vi "Configure Motor Controllers.vi"(8 "error in (no error)":errorcluster, 11 "Motion Magic Parameters":T1) -> (0 "error out":errorcluster)   [LabVIEW 2017, in "Drive Train.lvlib"]
uses:
  Drive Train.lvlib
  Controls/FGV Actions.ctl
  Controls/Motor Controllers Parameters.ctl
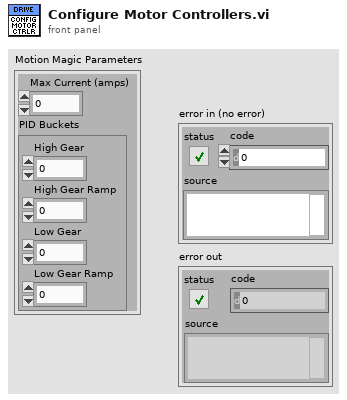
[diagram p1: front panel]
types:
  T1 = typedef "Drive Train.lvlib/Motor Controllers Parameters.ctl" = cluster{"Max Current (amps)":i32, "PID Buckets":cluster{"High Gear":i32, "High Gear Ramp":i32, "Low Gear":i32, "Low Gear Ramp":i32}}
  T2 = typedef "Drive Train.lvlib/FGV Actions.ctl" = enum16{"Get", "Set"}
  T3 = typedef "Drive Train.lvlib/Library Information.ctl" = cluster{"Right Motor Name":string, "Left Motor Name":string, "Current Control Mode":T4, "Motion Magic Parameters":T5, "Motor Controllers Parameters":T1}
  T4 = typedef "CTRE_Phoenix_MotorControl_ControlMode.ctl" = u16
  T5 = typedef "Drive Train.lvlib/Motion Magic Parameters.ctl" = cluster{"Native Units":dbl}
  T6 = typedef "WPI_MotorControlDeviceRef.ctl" = cluster{"DeviceStatus":errorcluster, "Type":T7, "PWM":cluster{"PWM Channel":T8, "DeadBand":T9}, "CAN":cluster{"Device Number":u8, "SetOutput VI Ref":variant, "GetOutput VI Ref":variant, "Enable VI Ref":variant, "Disable VI Ref":variant, "Data":variant}, "Invert":bool, "DIO PWM":cluster{"PWM \"Enable\" Channel":T8, "DIOChannel":T10, "PWM Rate":dbl}}
  T7 = typedef "WPI_MotorControlType.ctl" = enum16{"PWM", "CAN", "DIO PWM"}
  T8 = typedef "FPGA_DIOPWMChannel.ctl" = enum8{"PWM 0", "PWM 1", "PWM 2", "PWM 3", "PWM 4", "PWM 5", "PWM 6", "PWM 7", "PWM 8", "PWM 9", "PWM MXP 0", "PWM MXP 1", "PWM MXP 2", "PWM MXP 3", "PWM MXP 4", "PWM MXP 5", "PWM MXP 6", "PWM MXP 7", "PWM MXP 8", "PWM MXP 9", "Invalid"}
  T9 = typedef "WPI_PWMDeadband.ctl" = cluster{"Name":string, "maxPositivePwm":i32, "minPositivePwm":i32, "centerPwm":i32, "maxNegativePwm":i32, "minNegativePwm":i32, "angularRange":u16}
  T10 = typedef "FPGA_DIOChannel.ctl" = enum8{"DIO 0", "DIO 1", "DIO 2", "DIO 3", "DIO 4", "DIO 5", "DIO 6", "DIO 7", "DIO 8", "DIO 9", "DIO MXP 0", "DIO MXP 1", "DIO MXP 2", "DIO MXP 3", "DIO MXP 4", "DIO MXP 5", "DIO MXP 6", "DIO MXP 7", "DIO MXP 8", "DIO MXP 9", "DIO MXP 10", "DIO MXP 11", "DIO MXP 12", "DIO MXP 13", "DIO MXP 14", "DIO MXP 15", "SPI Port CS1", "SPI Port CS2", "SPI Port CS3", "SPI Port MISO", "SPI Port MOSI", "Invalid"}
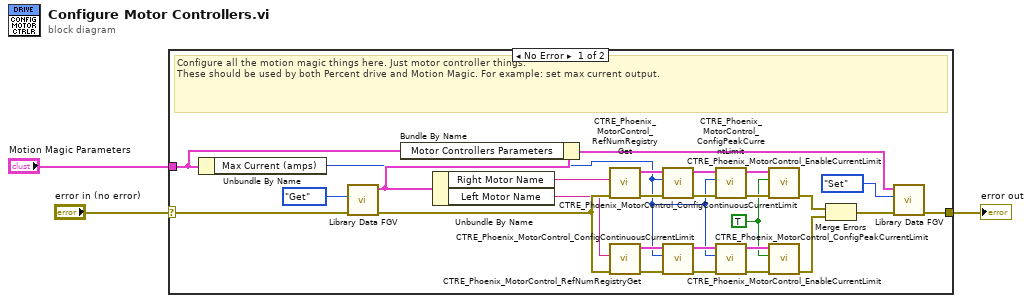
[diagram p0: block diagram]
diagram:
  n1 = case shown="No Error" "error in (no error)" {
    selector: "error in (no error)" -> [w30 w31]
    tunnel: [w23 w31] -> w2
    tunnel: "Motion Magic Parameters" -> [w4 _]
    frame No Error {
      w6 = TRUE ("Enable Current Limit?")
      # "Configure all the motion magic things here. Just motor controller things.\nThese should be used by both Percent drive and Motion Magic. For example: set max current output."
      n2 = Unbundle By Name(w4) -> ("Max Current (amps)"=w7:i32)
      n3 = call "Library Data FGV.vi"("error in (no error)"=w30, "FGV Actions"=FGV_Actions."Get") -> ("error out"=w28:errorcluster, "Library Information out"=w22:T3)  [unwired: 8 in]
      n4 = Bundle By Name(cluster=w22, "Motor Controllers Parameters"=w4) -> (w5:T3)
      n5 = Unbundle By Name(w22) -> ("Right Motor Name"=w26:string, "Left Motor Name"=w27:string)
      n6 = call <vilib>:"CTRE_Phoenix_MotorControl_RefNumRegistryGet.vi"("error in (no error)"=w28, "refnum name"=w26) -> ("error out"=w13:errorcluster, "PhoenixMotorControlDevRef"=w14:T6)  [unwired: 8 in]
      n7 = call <vilib>:"CTRE_Phoenix_MotorControl_RefNumRegistryGet.vi"("error in (no error)"=w28, "refnum name"=w27) -> ("error out"=w20:errorcluster, "PhoenixMotorControlDevRef"=w21:T6)  [unwired: 8 in]
      n8 = call <vilib>:"CTRE_Phoenix_MotorControl_ConfigContinuousCurrentLimit.vi"("error in (no error)"=w13, "Continuous Current Limit (Amps)"=w7, "PhoenixMotorControlDevRef"=w14) -> ("error out"=w11:errorcluster, "PhoenixMotorControlDevRef"=w12:T6)  [unwired: 7 in]
      n9 = call <vilib>:"CTRE_Phoenix_MotorControl_ConfigContinuousCurrentLimit.vi"("error in (no error)"=w20, "Continuous Current Limit (Amps)"=w7, "PhoenixMotorControlDevRef"=w21) -> ("error out"=w18:errorcluster, "PhoenixMotorControlDevRef"=w19:T6)  [unwired: 7 in]
      n10 = call <vilib>:"CTRE_Phoenix_MotorControl_ConfigPeakCurrentLimit.vi"("error in (no error)"=w11, "Peak Current (Amps)"=w7, "PhoenixMotorControlDevRef"=w12) -> ("error out"=w9:errorcluster, "PhoenixMotorControlDevRef"=w10:T6)  [unwired: 7 in]
      n11 = call <vilib>:"CTRE_Phoenix_MotorControl_ConfigPeakCurrentLimit.vi"("error in (no error)"=w18, "Peak Current (Amps)"=w7, "PhoenixMotorControlDevRef"=w19) -> ("error out"=w16:errorcluster, "PhoenixMotorControlDevRef"=w17:T6)  [unwired: 7 in]
      n12 = call <vilib>:"CTRE_Phoenix_MotorControl_EnableCurrentLimit.vi"("error in (no error)"=w9, "Enable Current Limit?"=w6, "PhoenixMotorControlDevRef"=w10) -> ("error out"=w8:errorcluster)  [unwired: 7 in, 1 out]
      n13 = call <vilib>:"CTRE_Phoenix_MotorControl_EnableCurrentLimit.vi"("error in (no error)"=w16, "Enable Current Limit?"=w6, "PhoenixMotorControlDevRef"=w17) -> ("error out"=w15:errorcluster)  [unwired: 7 in, 1 out]
      n14 = Merge Errors(w8, w15) -> (w24:errorcluster)
      n15 = call "Library Data FGV.vi"("error in (no error)"=w24, "FGV Actions"=FGV_Actions."Set", "Library Information in"=w5) -> ("error out"=w23:errorcluster)  [unwired: 7 in, 1 out]
    }
    frame Error {
    }
  }
  "error out" <- w2
